vi "Test RP VISA.vi"() -> ()   [LabVIEW 2015]
uses:
  RP Communicator VISA.lvclass
  RP Communicator VISA.lvclass/RP Communicator VISA.ctl
  Write Client type.vi
panel:
  out "error out 2":errorcluster
  out "error out":errorcluster
  out "Logic tag 2":u16
  out "IDN response 2":u32=1 format="0x%x (%d)"
  out "Logic tag":u16
  out "IDN response":u32=1 format="0x%x (%d)"
  in  "VISA resource name":refnum<visa-resource-name>
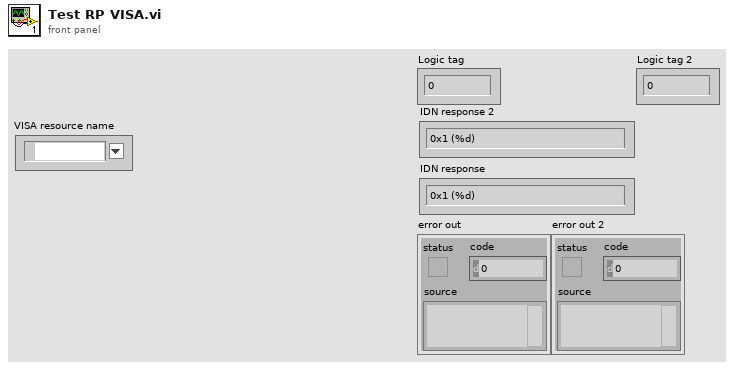
[diagram p1: front panel]
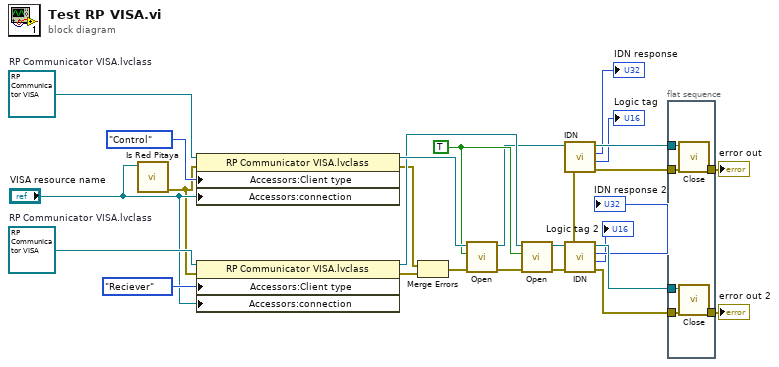
[diagram p0: block diagram]
diagram:
  w15 = TRUE ("Send \"Connect client\"")
  w24 = refnum<class "RP Communicator VISA.lvclass"> refnum  # RP Communicator VISA.lvclass
  w26 = refnum<class "RP Communicator VISA.lvclass"> refnum  # RP Communicator VISA.lvclass
  n1 = call "Is Red Pitaya.vi"("connection"="VISA resource name") -> ("Error Out"=w16:errorcluster)  [unwired: 6 in, 4 out]
  n2 = property class="RP Communicator VISA.lvclass"(reference=w26, error in=w16, "Accessors:Client type"=enum16{"Control", "Reciever", "Transmitter"}."Control" ("Client type"), "Accessors:connection"="VISA resource name") -> (reference out=w21:refnum<class "RP Communicator VISA.lvclass">, error out=w19:errorcluster)
  n3 = property class="RP Communicator VISA.lvclass"(reference=w24, error in=w16, "Accessors:Client type"=enum16{"Control", "Reciever", "Transmitter"}."Reciever" ("Client type"), "Accessors:connection"="VISA resource name") -> (reference out=w20:refnum<class "RP Communicator VISA.lvclass">, error out=w18:errorcluster)
  n4 = Merge Errors(w19, w18) -> (w17:errorcluster)
  n5 = call-dynamic "Open.vi"("error in (no error)"=w17, "Send \"Connect client\""=w15, "RP Communicator in"=w21) -> ("error out"=w10:errorcluster, "RP Communicator out"=w14:refnum<class "RP Communicator VISA.lvclass">)  [unwired: 7 in]
  n6 = call-dynamic "Open.vi"("error in (no error)"=w10, "Send \"Connect client\""=w15, "RP Communicator in"=w20) -> ("error out"=w6:errorcluster, "RP Communicator out"=w8:refnum<class "RP Communicator VISA.lvclass">)  [unwired: 7 in]
  n7 = call-dynamic "IDN.vi"("error in (no error)"=w6, "RP Communicator in"=w14) -> ("error out"=w9:errorcluster, "Logic tag"=→"Logic tag":u16, "IDN response"=→"IDN response":u32, "RP Communicator out"=w13:refnum<class "RP Communicator VISA.lvclass">)  [unwired: 6 in]
  n8 = call-dynamic "IDN.vi"("error in (no error)"=w6, "RP Communicator in"=w8) -> ("error out"=w5:errorcluster, "Logic tag"=→"Logic tag 2":u16, "IDN response"=→"IDN response 2":u32, "RP Communicator out"=w7:refnum<class "RP Communicator VISA.lvclass">)  [unwired: 6 in]
  n9 = flat-sequence {
    tunnel: w13 -> [w32]
    tunnel: w9 -> [w31]
    tunnel: w7 -> [w30]
    tunnel: w5 -> [w29]
    tunnel: [w28] -> w2
    tunnel: [w27] -> w1
    frame #0 {
      n10 = call-dynamic "Close.vi"("error in (no error)"=w31, "RP Communicator in"=w32) -> ("error out"=w28:errorcluster)  [unwired: 8 in, 1 out]
      n11 = call-dynamic "Close.vi"("error in (no error)"=w29, "RP Communicator in"=w30) -> ("error out"=w27:errorcluster)  [unwired: 8 in, 1 out]
    }
  }
  "error out" <- w2
  "error out 2" <- w1
